vi "Read Device Identification.vi"(7 "unit ID":u8, 8 "error in":errorcluster, 9 "read device ID code":T2, 10 "object ID":u8, 11 "Modbus slave in":refnum<class "Modbus Slave.lvclass">) -> (0 "error out":errorcluster, 2 "objects":T1[](array[typedef]) {"Object ID" format="%x"}, 3 "Modbus slave out":refnum<class "Modbus Slave.lvclass">)   [LabVIEW 2013, in "Modbus Library - Advance.lvlib" / "Modbus Slave.lvclass"]
doc: "Reads Modbus object information stored on the device. This can include basic information, like manufacturer, additional standard items, or model-specific extended items. This function may take a large amount of time to execute, as it requires the transfer of a large quantity of binary data. Even on TCP/IP, this function is limited by the maximum defined size of a Modbus protocol data unit."
uses:
  Modbus Slave.lvclass
  Master Function Definition/Read Device ID code.ctl
  Data Model/Identification Parameters.ctl
  Modbus Slave.lvclass/Modbus Slave.ctl
  Standard Data Model/Standard Data Model.lvclass
  Data Model/Device Data Model.lvclass
  Super Data Model/Super Data Model.lvclass
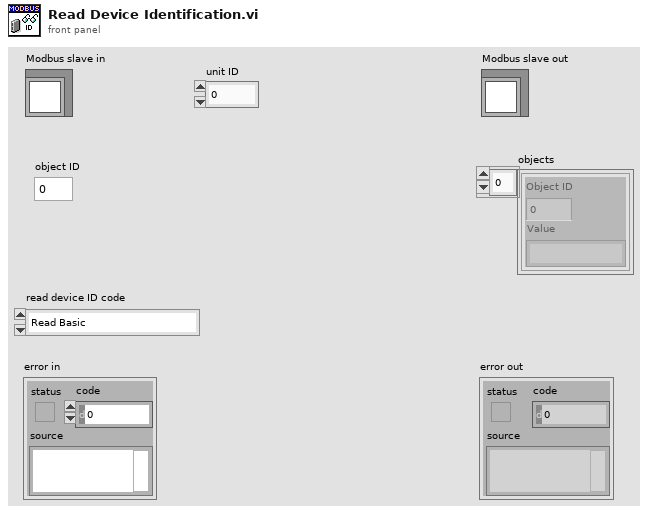
[diagram p1: front panel]
types:
  T1 = typedef "Modbus Library - Advance.lvlib/Device Data Model.lvclass/Identification Parameters.ctl" = cluster{"Object ID":u8, "Value":string}
  T2 = typedef "Modbus Library - Advance.lvlib/Device Data Model.lvclass/Read Device ID code.ctl" = enum8{"Read Basic", "Read Regular", "Read Extended", "Read Specific"}
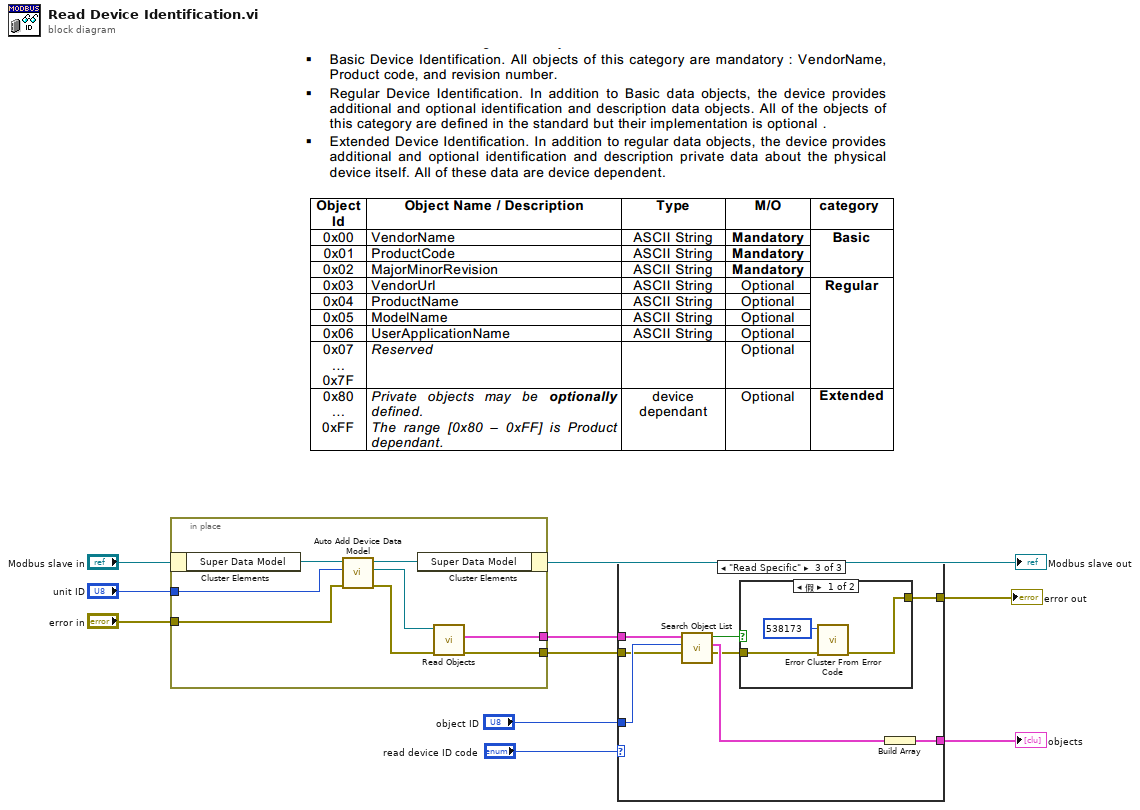
[diagram p0: block diagram]
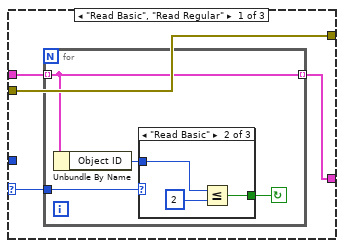
[diagram p2: hidden frame]
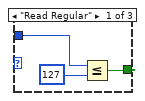
[diagram p3: hidden frame]
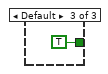
[diagram p4: hidden frame]
diagram:
  n1 = in-place {
    in-place-border: [w18] -> w5
    in-place-border: [w17] -> w2
    in-place-border: "error in" -> [w13]
    in-place-border: "unit ID" -> [w14]
    n2 = in-place-cluster #1("Modbus slave in") -> ("Super Data Model"=w16:refnum<class "Super Data Model.lvclass">)
    n3 = call "Auto Add Device Data Model.vi"("error in"=w13, "unit ID"=w14, "Super Data Model in"=w16) -> ("error out"=w11:errorcluster, "device data model"=w12:refnum<class "Standard Data Model.lvclass">, "Super Data Model out"=w15:refnum<class "Super Data Model.lvclass">)  [unwired: 6 in]
    n4 = in-place-cluster #1("Super Data Model"=w15) -> (→"Modbus slave out":refnum<class "Modbus Slave.lvclass">)
    n5 = call-dynamic "Read Objects.vi"("error in"=w11, "device data model in"=w12) -> ("error out"=w17:errorcluster, "Objects"=w18:T1[])  [unwired: 7 in, 1 out]
  }
  n6 = case shown="\"Read Specific\"" "read device ID code" {
    selector: "read device ID code" -> [w19 _ _]
    tunnel: w5 -> [w21 w34 w42]
    tunnel: w2 -> [w22 w35 w37]
    tunnel: "object ID" -> [_ _ w41]
    tunnel: [w20 w34 w38] -> w8
    tunnel: [w22 w35 w36] -> w7
    frame "Read Basic", "Read Regular" {
      n7 = for {
        tunnel: w21 -> [w24] mode=indexing
        tunnel: [w24] -> w20 mode=indexing
        tunnel: w19 -> [w26]
        stop <- w25 continue-if-true
        n8 = Unbundle By Name(w24) -> ("Object ID"=w23:u8)
        n9 = case shown="\"Read Basic\"" w26 {
          tunnel: w23 -> [w29 w32 _]
          tunnel: [w27 w30 TRUE] -> w25
          frame "Read Regular" {
            n10 = Less Or Equal?(x=w29, y=u8 127) -> (x <= y?=w27:bool)
          }
          frame "Read Basic" {
            n11 = Less Or Equal?(x=w32, y=u8 2) -> (x <= y?=w30:bool)
          }
          frame Default {
          }
        }
      }
    }
    frame "Read Extended" {
    }
    frame "Read Specific" {
      n12 = call "Search Object List.vi"("Object ID"=w41, "Objects"=w42) -> ("Object"=w39:T1, "Found?"=w40:bool)  [unwired: 7 in, 1 out]
      n13 = case shown="假" w40 {
        tunnel: w37 -> [w44 w46]
        tunnel: [w45 w46] -> w36
        frame False {
          n14 = call <vilib>:"Error Cluster From Error Code.vi"("error in (no error)"=w44, "error code (0)"=538173) -> ("error out"=w45:errorcluster)  [unwired: 7 in]
        }
        frame True {
        }
      }
      n15 = Build Array(w39) -> (w38:T1[])
    }
  }
  "error out" <- w7
  "objects" <- w8
